vi "UV-VIS PrepareAcquisition.vi"(3 "error in (no error)":errorcluster, 5 "Detector in":refnum<class "CCD_camera.lvclass">) -> (0 "error out":errorcluster, 1 "DLL error code":u32, 2 "Detector out":refnum<class "CCD_camera.lvclass">)   [LabVIEW 2020, in "CCD_camera.lvclass"]
doc: "The <B>PrepareAcquisition</B> function reads the current acquisition setup and allocates and clears any memory that will be used during the acquisition. The function call is not required as it will be called automatically by the <B>StartAcquisition</B> function if it has not already been called externally. However for long kinetic series acquisitions the time to allocate and clear any memory can be quite long which can result in a long delay between calling <B>StartAcquisition</B> and the acquisition actually commencing. Calling <B>PrepareAcquisition</B> first will reduce this delay in the <B>StartAcquisition</B> call.\n\n<B>Error codes:</B>\nDRV_SUCCESS - Acquisition prepared.\nDRV_NOT_INITIALIZED - System not initialized.\nDRV_ACQUIRING - Acquisition in progress.\nDRV_VXDNOTINSTALLED - VxD not loaded.\nDRV_ERROR_ACK - Unable to communicate with card.\nDRV_INIERROR - Error reading \"DETECTOR.INI\".\nDRV_ACQUISITION_ERRORS - Acquisition settings invalid.\nDRV_ERROR_PAGELOCK - Unable to allocate memory.\nDRV_INVALID_FILTER - Filter not available for current acquisition.\nDRV_IOCERROR - Integrate On Chip setup error."
uses:
  CCD_camera.lvclass
  C:/dev/TRANCON/Classes/Detector/Detector.lvclass
  Detector.lvclass/Detector.ctl
  Detector.lvclass
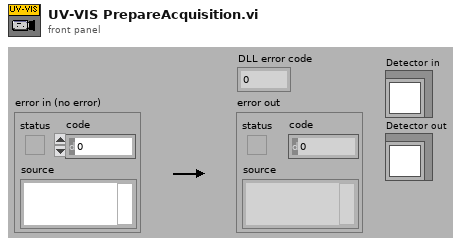
[diagram p1: front panel]
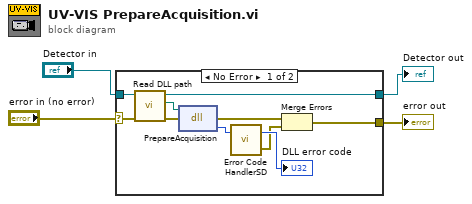
[diagram p0: block diagram]
diagram:
  n1 = case shown="No Error" "error in (no error)" {
    selector: "error in (no error)" -> [w12 w16]
    tunnel: [w8 w16] -> w3
    tunnel: "Detector in" -> [w6 w15]
    tunnel: [w5 w15] -> w1
    frame No Error {
      n2 = call "Read DLL path.vi"("error in (no error)"=w12, "Detector in"=w6) -> ("error out"=w10:errorcluster, "DLL path"=w11:path, "Detector out"=w5:refnum<class "CCD_camera.lvclass">)  [unwired: 7 in]
      n3 = dll-call lib="S:/TRANCON/DLL/Atmcd32d.dll" fn="PrepareAcquisition"(path in=w11, error in=w10) -> (error out=w7:errorcluster, "return type"=w14:u32)  [unwired: 1 in, 1 out]
      n4 = call "Error Code HandlerSD.vi"("DLL error code"=w14) -> ("error out"=w9:errorcluster, "dup DLL error code"=→"DLL error code":u32)  [unwired: 1 in]
      n5 = Merge Errors(w7, w9) -> (w8:errorcluster)
    }
    frame Error {
    }
  }
  "error out" <- w3
  "Detector out" <- w1
